vi "CommandServoPosition.vi"(8 "Error in":errorcluster, 10 "Suggested Rudder Setpoint":T1 min=-1.0 max=1.0 scale=1.0..-1.0, 11 "PWM Ref In":T2) -> (0 "Error out":errorcluster, 3 "duty cycle [%]":dbl)   [LabVIEW 2013]
uses:
  <vilib>/myRIO/Instrument Drivers/Onboard IO/PWM/typedefs/PWM Reference.ctl
  <vilib>/myRIO/Common/Instrument Driver Framework/Utilities/typedefs/myRIO Generic Hardware Reference.ctl
  <vilib>/myRIO/Common/Instrument Driver Framework/Utilities/typedefs/Hardware Version Enum.ctl
  <vilib>/myRIO/Common/Instrument Driver Framework/Utilities/typedefs/myRIO v1.0 Reference.ctl
  <vilib>/myRIO/Common/Instrument Driver Framework/Utilities/typedefs/Generic FPGA Reference.ctl
  <vilib>/myRIO/Common/Instrument Driver Framework/myRIO v1.0/PWM/typedefs/PWM Channels Enum.ctl
  <vilib>/myRIO/Instrument Drivers/Onboard IO/PWM/typedefs/PWM Configuration.ctl
  Data/TypeDefs/Rudder Set Suggestions.ctl
  <vilib>/myRIO/Common/Instrument Driver Framework/myRIO v1.0/PWM/vis/myRIO v1.0 Write PWM.vi
  <vilib>/Utility/error.llb/Error Cluster From Error Code.vi
  <vilib>/myRIO/Instrument Drivers/Onboard IO/PWM/PWM.lvlib
panel:
  out "offset [%FS]":dbl
  in  "null offset":bool
  out "pulse width [ms]":dbl=1.5
  in  "freq [Hz]":dbl=50.0
  in  "position [%FS]":dbl(slide) scale=-200.0..200.0
  # "Default settings from MyRIO example servo command code"
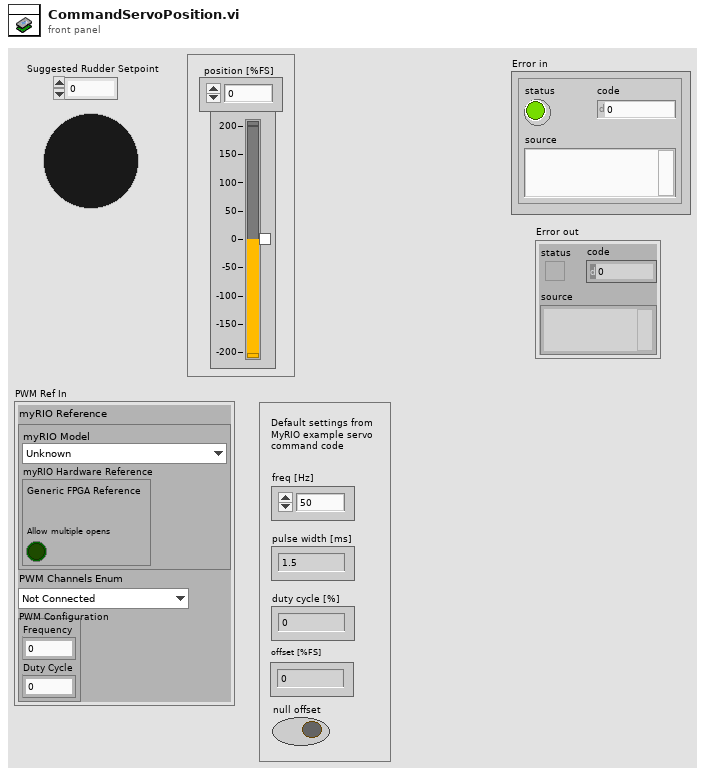
[diagram p1: front panel]
types:
  T1 = typedef "Rudder Set Suggestions.ctl" = dbl
  T2 = typedef "PWM.lvlib/PWM Reference.ctl" = cluster{"myRIO Reference":T3, "PWM Channels Enum":T7, "PWM Configuration":T8}
  T3 = typedef "myRIO Generic Hardware Reference.ctl" = cluster{"myRIO Model":T4, "myRIO Hardware Reference":T5}
  T4 = typedef "Hardware Version Enum.ctl" = enum16{"Unknown", "myRIO-1900", "myRIO-1950"}
  T5 = typedef "myRIO v1.0 Reference.ctl" = cluster{"Generic FPGA Reference":T6, "Allow multiple opens":bool}
  T6 = typedef "Generic FPGA Reference.ctl" = refnum<k20>
  T7 = typedef "PWM Channels Enum.ctl" = enum16{"Not Connected", "C/PWM0", "C/PWM1", "A/PWM0", "A/PWM1", "A/PWM2", "B/PWM0", "B/PWM1", "B/PWM2"}
  T8 = typedef "PWM.lvlib/PWM Configuration.ctl" = cluster{"Frequency":dbl, "Duty Cycle":dbl}
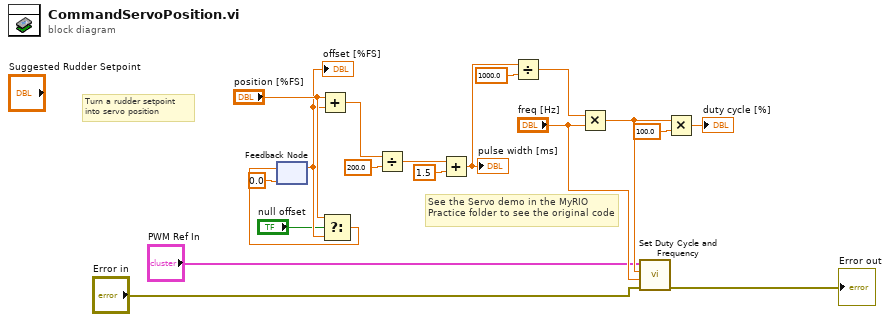
[diagram p0: block diagram]
diagram:
  # "Turn a rudder setpoint\ninto servo position"
  # "See the Servo demo in the MyRIO Practice folder to see the original code"
  n1 = feedback #1(0.0 ("position [%FS]")) -> (w13:dbl)
  "offset [%FS]" <- w13
  n2 = Add(x="position [%FS]", y=w13) -> (x+y=w12:dbl)
  n3 = Select(t="position [%FS]", s="null offset", f=w13) -> (s? t:f=w11:dbl)
  n4 = feedback-in #1(w11) -> ()
  n5 = Divide(x=w12, y=200.0) -> (x/y=w5:dbl)
  n6 = Add(x=w5, y=1.5) -> (x+y=w7:dbl)
  "pulse width [ms]" <- w7
  n7 = Divide(x=w7, y=1000.0) -> (x/y=w15:dbl)
  n8 = Multiply(x=w15, y="freq [Hz]") -> (x*y=w18:dbl)
  n9 = call <vilib>:"Set Duty Cycle and Frequency.vi"("error in (no error)"="Error in", "Frequency (Hz)"="freq [Hz]", "Duty Cycle (0-1)"=w18, "PWM Ref In"="PWM Ref In") -> ("error out"=→"Error out":errorcluster)  [unwired: 5 in, 1 out]
  n10 = Multiply(x=w18, y=100.0) -> (x*y=→"duty cycle [%]":dbl)
